vi "dfd_FXP Decimation Simu.vi"(0 "signal in":i64[](array[numeric]), 2 "PROD2SUM":i16, 3 "init?":bool, 7 "decimation factor":i32, 9 "coef":i64[](array[numeric]), 11 "FXPMRateSimState in":T1, 12 "#taps per phase":i32, 13 "output phase":i32) -> (4 "signal out":i64[](array[numeric]), 15 "FXPMRateSimState out":T1)   [LabVIEW 2017, in "NI_DigFilter_FXP.lvlib"]
uses:
  <vilib>/addons/Digital Filter Design/NI_DigFilter_FXP.lvlib
  <vilib>/addons/Digital Filter Design/_Objects.llb/dfd_FXP MRate Simu State.ctl
  <vilib>/addons/Digital Filter Design/_Objects.llb/dfd_Integer I160.ctl
  <vilib>/addons/Digital Filter Design/_Objects.llb/dfd_Index Config.ctl
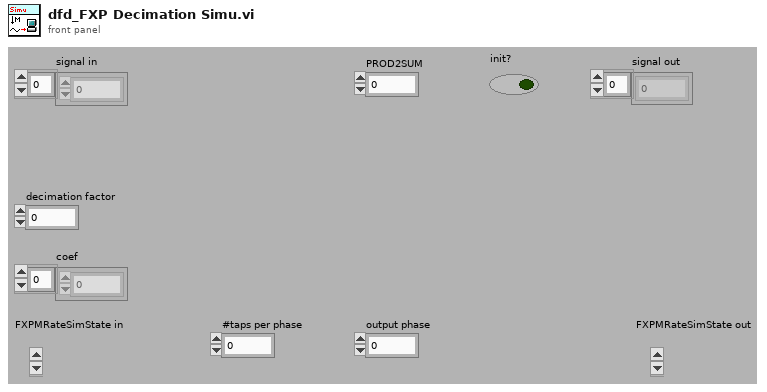
[diagram p1: front panel]
types:
  T1 = typedef "dfd_FXP MRate Simu State.ctl" = cluster{"acc1":T2[], "acc2":T2[], "FIR state":i64[], "next phase":i32}
  T2 = typedef "dfd_Integer I160.ctl" = cluster{"Hi [I32]":i32, "Lo3 [U32]":u32, "Lo2 [U32]":u32, "Lo1 [U32]":u32, "Lo0 [U32]":u32}
  T3 = typedef "dfd_Index Config.ctl" = cluster{"start":i32, "stepsize":i32}
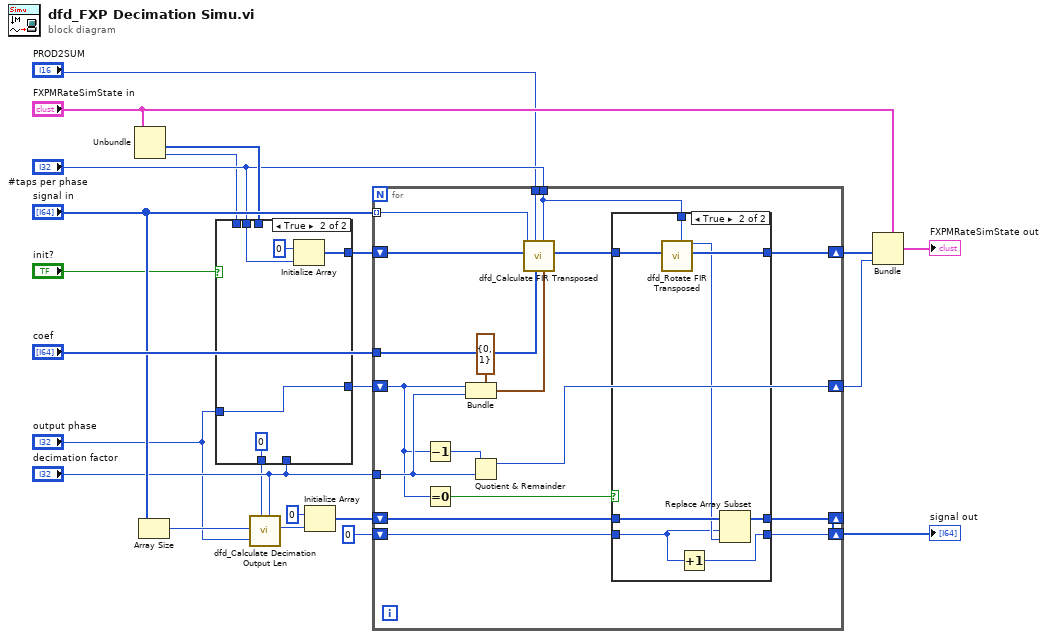
[diagram p0: block diagram]
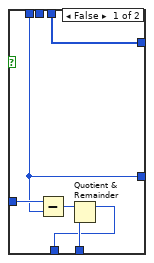
[diagram p2: hidden frame]
diagram:
  n1 = Unbundle("FXPMRateSimState in") -> ("FIR state"=w10:i64[], "next phase"=w8:i32)  [unwired: 2 out]
  n2 = Array Size(array="signal in") -> (size(s)=w20:i32)
  n3 = case shown="True" "init?" {
    tunnel: [w25 w32] -> w17
    tunnel: "#taps per phase" -> [_ w29]
    tunnel: "output phase" -> [w24 w31]
    tunnel: [w23 w31] -> w13
    tunnel: [w26 0] -> w12
    tunnel: "decimation factor" -> [w27 _]
    tunnel: w10 -> [w25 _]
    tunnel: w8 -> [w23 _]
    frame False {
      n4 = Subtract(x=w24, y=w23) -> (x-y=w28:i32)
      n5 = Quotient & Remainder(x=w28, y=w27) -> (x-y*floor(x/y)=w26:i32)  [unwired: 1 out]
    }
    frame True {
      n6 = Initialize Array(i64 0, w29) -> (w32:i64[])
    }
  }
  n7 = call <vilib>:"dfd_Calculate Decimation Output Len.vi"("factor"="decimation factor", "output phase"="output phase", "current phase"=w12, "signal in len"=w20) -> ("signal out len"=w14:i32)  [unwired: 7 out]
  n8 = Initialize Array(i64 0 ("element"), w14) -> (w11:i64[])
  n9 = for {
    tunnel: "signal in" -> [w35] mode=indexing
    shift-right: [w45] -> w6
    shift-left: w17 -> [w51]
    tunnel: "coef" -> [w50]
    shift-right: [w47] -> w5
    shift-left: w13 -> [w41]
    tunnel: "decimation factor" -> [w42]
    tunnel: "#taps per phase" -> [w37]
    shift-right: [w43] -> w1
    shift-left: w11 -> [w44]
    shift-right: [w38] -> _
    shift-left: 0 ("element") -> [w39]
    tunnel: "PROD2SUM" -> [w34]
    n10 = Decrement(x=w41) -> (x-1=w36:i32)
    n11 = Equal To 0?(x=w41) -> (x = 0?=w40:bool)
    n12 = Bundle(cluster=T3 {"start"=0, "stepsize"=1} ("state idx"), "start"=w41, "stepsize"=w42) -> (w48:T3)
    n13 = Quotient & Remainder(x=w36, y=w42) -> (x-y*floor(x/y)=w47:i32)  [unwired: 1 out]
    n14 = call <vilib>:"dfd_Calculate FIR Transposed.vi"("coef idx"=w48, "#taps per phase"=w37, "coef"=w50, "Fwldiff"=w34, "state in"=w51, "x"=w35) -> ("state out"=w46:i64[])  [unwired: 2 in, 3 out]
    n15 = case shown="True" w40 {
      tunnel: w46 -> [w54 w62]
      tunnel: [w54 w61] -> w45
      tunnel: w37 -> [_ w60]
      tunnel: w44 -> [w53 w59]
      tunnel: [w53 w58] -> w43
      tunnel: w39 -> [w52 w55]
      tunnel: [w52 w56] -> w38
      frame False {
      }
      frame True {
        n16 = call <vilib>:"dfd_Rotate FIR Transposed.vi"("#taps per phase"=w60, "state in"=w62) -> ("state out"=w61:i64[], "y"=w57:i64)  [unwired: 1 in, 7 out]
        n17 = Increment(x=w55) -> (x+1=w56:i32)
        n18 = Replace Array Subset(array=w59, new element=w57, index=w55) -> (w58:i64[])
      }
    }
  }
  "signal out" <- w1
  n19 = Bundle(cluster="FXPMRateSimState in", "FIR state"=w6, "next phase"=w5) -> (→"FXPMRateSimState out":T1)  [unwired: 2 out]
